vi "Initialize Serial Communications.vi"(0 "Serial Port":refnum<visa-resource-name>="COM32", 5 "timeout (msec)":u32=1000, 7 "Baud Rate":u32=115200, 9 "Buffer Size":u32=5000, 11 "error in":errorcluster) -> (4 "Serial Port Out":refnum<visa-resource-name>="COM32", 15 "error out":errorcluster)   [LabVIEW 2017]
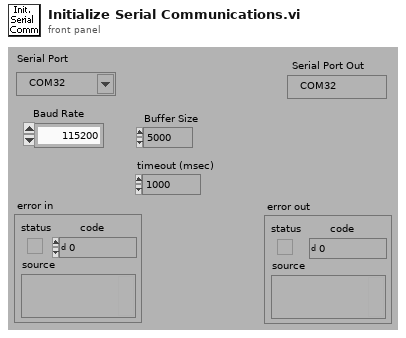
[diagram p1: front panel]
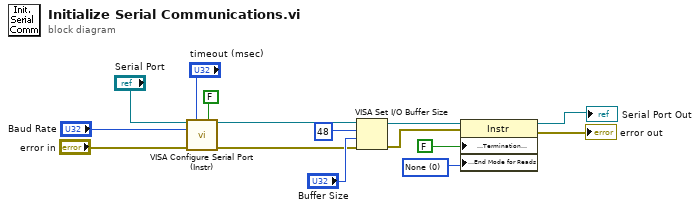
[diagram p0: block diagram]
diagram:
  w3 = u16 0 items=["None", "LastBit", "TermChar"] ("Serial Settings:Serial End Mode for Reads")
  n1 = call <vilib>:"VISA Configure Serial Port (Instr).vi"("VISA resource name"="Serial Port", "timeout (10sec)"="timeout (msec)", "Enable Termination\nChar (T)"=FALSE ("Message Based Settings:Termination Character Enable"), "baud rate (9600)"="Baud Rate", "error in (no error)"="error in") -> ("VISA resource name out"=w13:refnum<visa-resource-name>, "error out"=w1:errorcluster)  [unwired: 9 in]
  n2 = VISA Set I/O Buffer Size(VISA resource name=w13, mask (16)=u16 48, size (4096)="Buffer Size", error in (no error)=w1) -> (VISA resource name out=w8:refnum<visa-resource-name>, error out=w6:errorcluster)
  n3 = property class="Instr"(reference=w8, error in=w6, "Message Based Settings:Termination Character Enable"=FALSE, "Serial Settings:End Mode for Reads"=w3) -> (reference out=→"Serial Port Out":refnum<visa-resource-name>, error out=→"error out":errorcluster)
